vi "RT Loop - Motion and Lighting.vi"(8 "error in (no error)":errorcluster, 9 "FPGA VI Reference":T2, 11 "Message Queues out":T1) -> ()   [LabVIEW 2018]
doc: "Executes the sequence sent from the main UI."
uses:
  Globals/Global - All RT Loop Stop.vi
  support/Message Queue/Message Queue.lvlib
  support/Message Queue/Message Cluster (string).ctl
  controls/FPGA VI Reference.ctl
  support/Message Queue/Message (enum).ctl
  support/Message Queue/Message Cluster (enum).ctl
  support/Message Queue/All Message Queues (RT).ctl
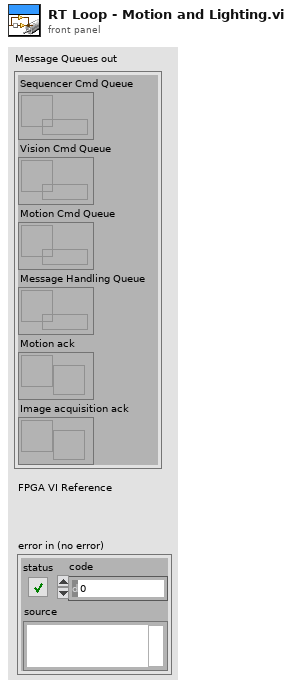
[diagram p1: front panel]
types:
  T1 = typedef "Message Queue.lvlib/All Message Queues (RT).ctl" = cluster{"Sequencer Cmd Queue":refnum<queue>, "Vision Cmd Queue":refnum<queue>, "Motion Cmd Queue":refnum<queue>, "Message Handling Queue":refnum<queue>, "Motion ack":refnum<notifier>, "Image acquisition ack":refnum<notifier>}
  T2 = typedef "FPGA VI Reference.ctl" = refnum<k20>
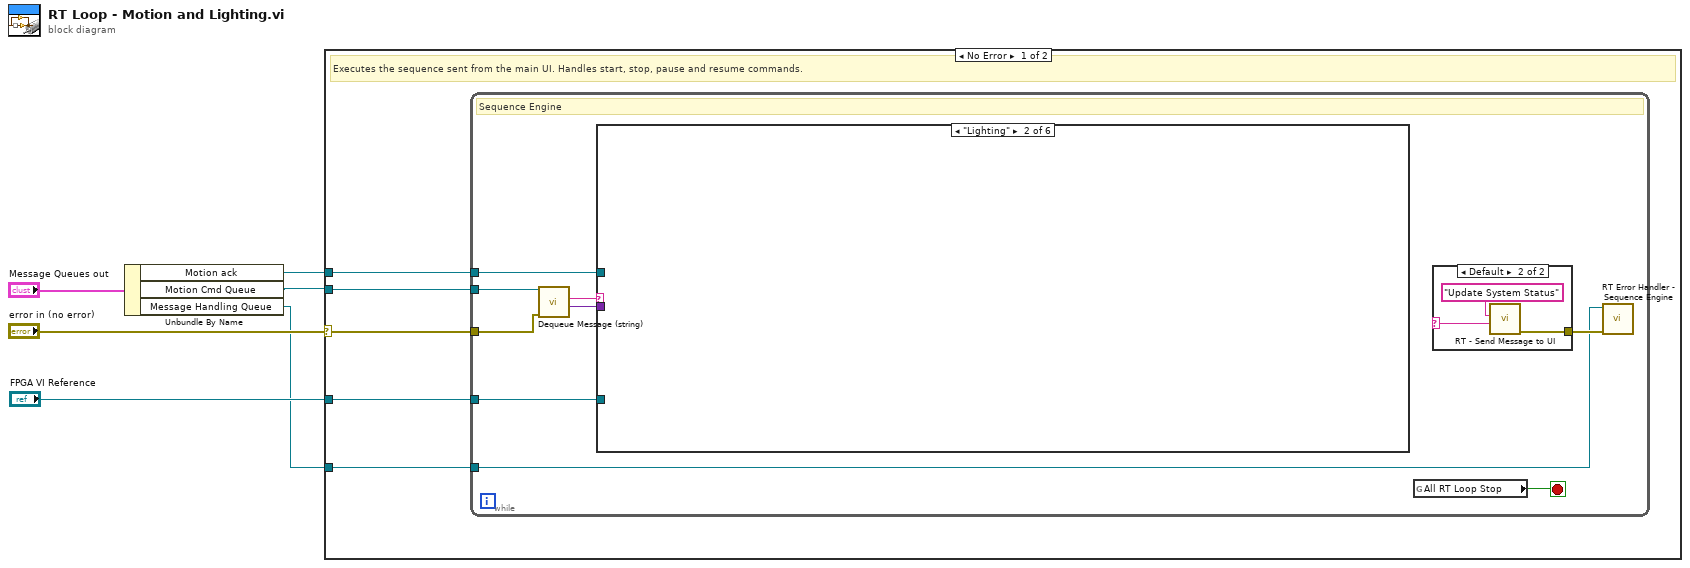
[diagram p0: block diagram]
diagram:
  n1 = Unbundle By Name("Message Queues out") -> ("Motion ack"=w1:refnum<notifier>, "Motion Cmd Queue"=w3:refnum<queue>, "Message Handling Queue"=w2:refnum<queue>)
  n2 = case shown="No Error" "error in (no error)" {
    selector: "error in (no error)" -> [w8 _]
    tunnel: w2 -> [w11 _]
    tunnel: w3 -> [w10 _]
    tunnel: "FPGA VI Reference" -> [w9 _]
    tunnel: w1 -> [w7 _]
    frame No Error {
      # "Executes the sequence sent from the main UI. Handles start, stop, pause and resume commands."
      n3 = while "Sequence Engine" {
        tunnel: w10 -> [w16]
        tunnel: w9 -> [w20]
        tunnel: w11 -> [w18]
        tunnel: w8 -> [w15]
        tunnel: w7 -> [w12]
        stop <- w17 stop-if-true
        # "Sequence Engine"
        n4 = call "Dequeue Message (string).vi"("error in (no error)"=w15, "Message Queue"=w16) -> ("Message Data"=w13:variant, "Message"=w14:string)  [unwired: 6 in, 2 out]
        n5 = case shown="\"Lighting\"" w14 {
          tunnel: w20 -> [_ _ _ _ _ _]
          tunnel: w13 -> [_ _ _ _ _ _]
          tunnel: w12 -> [_ _ _ _ _ _]
          frame "Initialize" {
          }
          frame "Lighting" {
          }
          frame "Vacuum actuator" {
          }
          frame "Actuator 1" {
          }
          frame "Actuator 2" {
          }
          frame "Stop" {
          }
        }
        n6 = global read "Global - All RT Loop Stop.vi" "All RT Loop Stop"() -> (w17:bool)
        n7 = case shown="Default" {
          selector: _ -> [_ w22]
          tunnel: [w21 w23] -> w19
          frame "" {
            # "Blank. Send nothing."
          }
          frame Default {
            n8 = call "RT - Send Message to UI.vi"("Message Data"=w22, "Message"="Update System Status") -> ("error out"=w23:errorcluster)  [unwired: 9 in]
          }
        }
        n9 = call "RT Error Handler - Sequence Engine.vi"("error in (no error)"=w19, "Message Queue"=w18) -> ()  [unwired: 9 in, 1 out]
      }
    }
    frame Error {
      # "Input Error. Do nothing."
    }
  }
